vi "Add.vi"(1 "Vec2 b in":refnum<class "Vector2.lvclass">, 2 "Vec2 a in":refnum<class "Vector2.lvclass">) -> (0 "Vec2 out":refnum<class "Vector2.lvclass">)   [LabVIEW 2022 SP3, in "Vector2.lvclass"]
uses:
  Vector2.lvclass
  Vector2.lvclass/Vector2.ctl
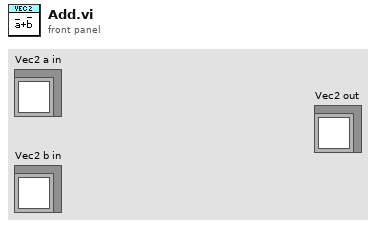
[diagram p1: front panel]
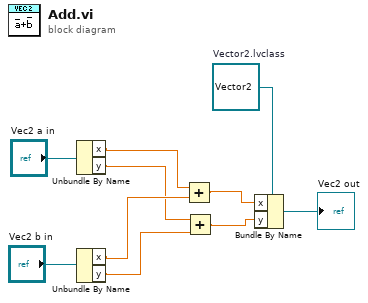
[diagram p0: block diagram]
diagram:
  w4 = refnum<class "Vector2.lvclass"> refnum  # Vector2.lvclass
  n1 = Unbundle By Name("Vec2 a in") -> ("x"=w8:sgl, "y"=w6:sgl)
  n2 = Unbundle By Name("Vec2 b in") -> ("x"=w7:sgl, "y"=w5:sgl)
  n3 = Add(x=w8, y=w7) -> (x+y=w3:sgl)
  n4 = Add(x=w6, y=w5) -> (x+y=w2:sgl)
  n5 = Bundle By Name(cluster=w4, "x"=w3, "y"=w2) -> (→"Vec2 out":refnum<class "Vector2.lvclass">)
